vi "LC2_send_command.vi"() -> ()   [LabVIEW 2018]
panel:
  out "Reply 2":string
  out "Reply":string
  in  "Send Command":bool
  in  "Stop Button":bool
  in  "Command":string="Bob"
  in  "LC2 IP Address":string="10.0.94.137"
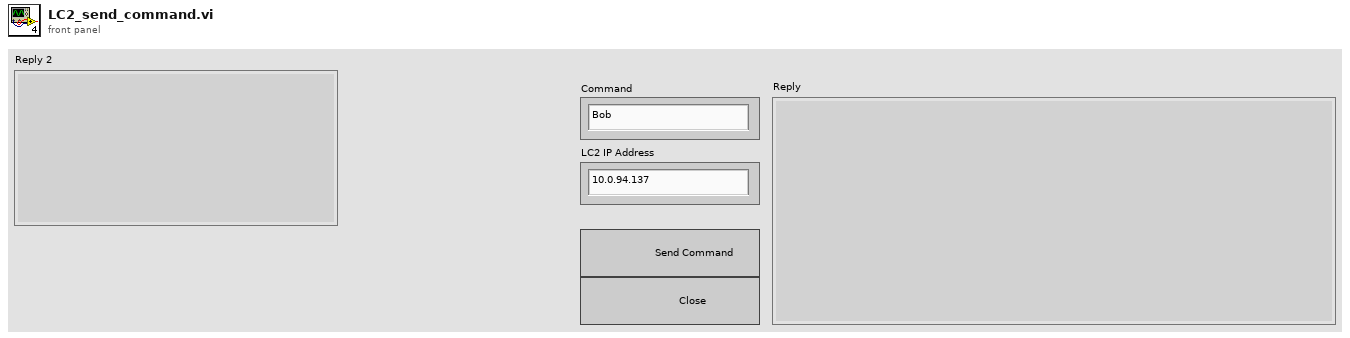
[diagram p1: front panel]
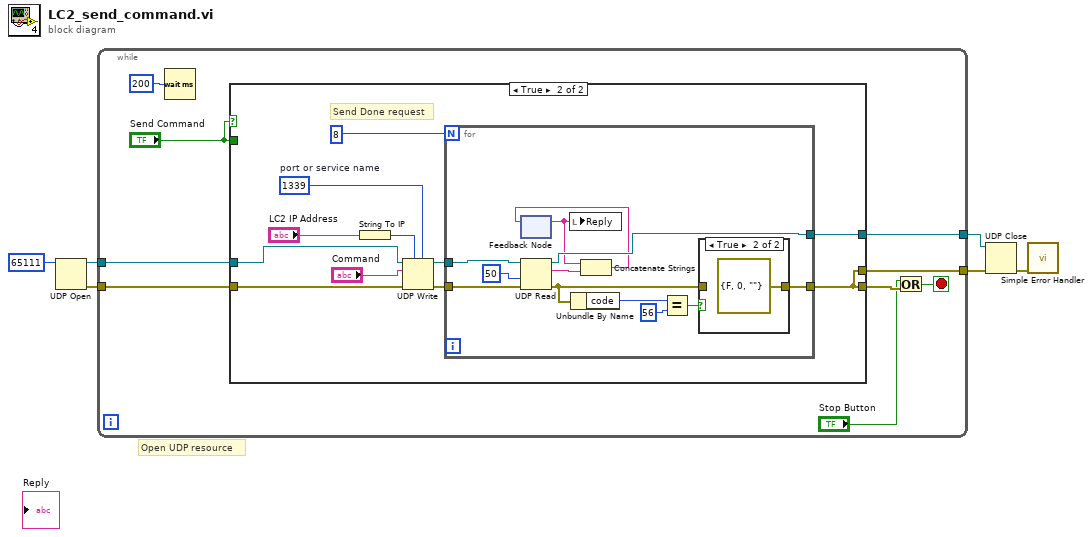
[diagram p0: block diagram]
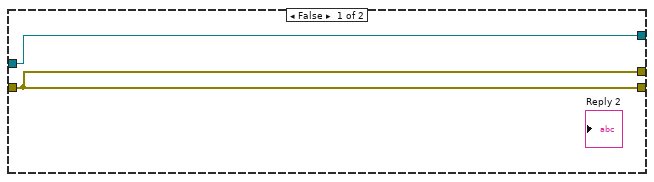
[diagram p2: hidden frame]
diagram:
  # "Open UDP resource"
  n1 = UDP Open(11:u16 65111 ("port")) -> (port=w6:refnum<k16>, 0:w5:errorcluster)  [unwired: 4 in, 1 out]
  n2 = while {
    tunnel: w6 -> [w14]
    tunnel: w5 -> [w13]
    tunnel: [w11] -> w3
    tunnel: [w10] -> w2
    stop <- w8 stop-if-true
    n3 = Wait (ms)(milliseconds to wait=u32 200) -> ()  [unwired: 1 out]
    n4 = case shown="True" "Send Command" {
      tunnel: w14 -> [w16 w28]
      tunnel: w13 -> [w17 w27]
      tunnel: [w17 w18] -> w12
      tunnel: [w16 w19] -> w11
      tunnel: [w17 w18] -> w10
      tunnel: "Send Command" -> [_ _]
      frame False {
      }
      frame True {
        w21 = u16 1339  # port or service name
        # "Send Done request"
        n5 = String To IP(1:"LC2 IP Address") -> (0:w25:u32)
        n6 = UDP Write(address=w25, port or service name=w21, connection ID=w28, data in="Command", 8:w27) -> (error out=w23:errorcluster, 3:w24:refnum<k16>)  [unwired: 1 in]
        n7 = for {
          N: 8 -> [_]
          tunnel: w24 -> [w40]
          tunnel: w23 -> [w39]
          tunnel: [w29] -> w18
          tunnel: [w37] -> w19
          n8 = feedback #1() -> (w34:string)  [unwired: 1 in]
          n9 = UDP Read(connection ID=w40, timeout ms (25000)=50, 8:w39) -> (data out=w36:string, error out=w30:errorcluster, 3:w37:refnum<k16>)  [unwired: 1 in, 2 out]
          n10 = local write "Reply"(w34) -> ()
          n11 = Unbundle By Name(w30) -> ("code"=w33:i32)
          n12 = Concatenate Strings(w34, w36) -> (w35:string)
          n13 = feedback-in #1(w35) -> ()
          n14 = Equal?(x=w33, y=56) -> (x = y?=w31:bool)
          n15 = case shown="True" w31 {
            tunnel: w30 -> [w41 _]
            tunnel: [w41 errorcluster {"status"=FALSE, "code"=0, "source"=""} ("error out")] -> w29
            frame False {
            }
            frame True {
            }
          }
        }
      }
    }
    n16 = Or(x="Stop Button", y=w12) -> (x .or. y?=w8:bool)
  }
  n17 = UDP Close(connection ID=w3, 8:w2) -> (error out=w1:errorcluster)  [unwired: 1 out]
  n18 = call <vilib>:"Simple Error Handler.vi"("error in (no error)"=w1) -> ()  [unwired: 4 in, 5 out]
